vi "FPGA - Download (ECAT).vi"(8 "error in (no error)":errorcluster, 11 "Node Ptr":u64 format="%.0x") -> (0 "error out":errorcluster)   [LabVIEW 2016, in "Scan Engine Custom Device.lvlib"]
uses:
  Scan Engine Custom Device.lvlib
  Type Defs/FPGA Target.ctl
panel:
  in  "Tag":string
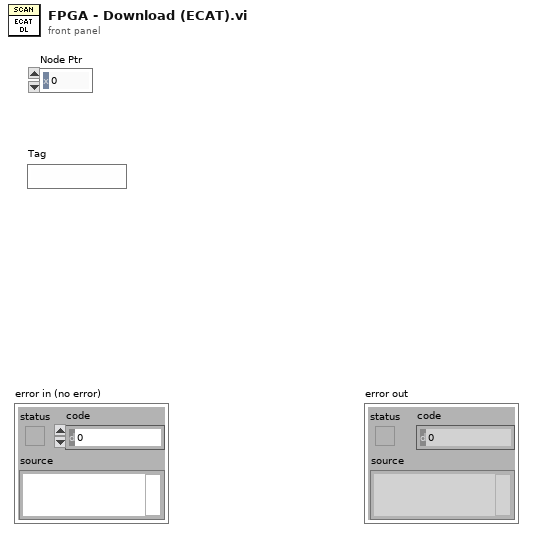
[diagram p1: front panel]
types:
  T1 = typedef "Scan Engine Custom Device.lvlib/FPGA Target.ctl" = enum16{"Local", "EtherCAT"}
  T2 = typedef "Custom Device API.lvlib/Custom Device Item Ref.ctl" = u64
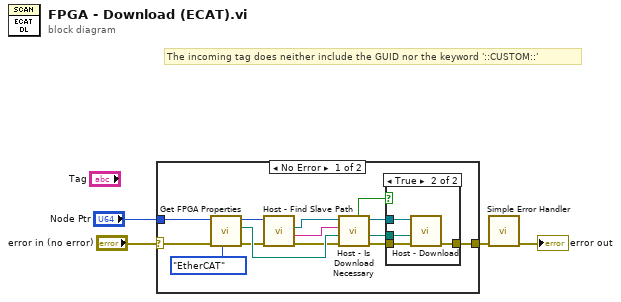
[diagram p0: block diagram]
diagram:
  # "The incoming tag does neither include the GUID nor the keyword '::CUSTOM::'"
  n1 = case shown="No Error" "error in (no error)" {
    selector: "error in (no error)" -> [w7 w24]
    tunnel: "Node Ptr" -> [w5 _]
    tunnel: [w6 w24] -> w2
    frame No Error {
      n2 = call "Get FPGA Properties.vi"("FPGA Target"=FPGA_Target."EtherCAT", "error in (no error)"=w7, "Item Ref in"=w5) -> ("error out"=w11:errorcluster, "Bitfile Path"=w13:path, "Item Ref out"=w12:T2)  [unwired: 5 in, 1 out]
      n3 = call "Host - Find Slave Path.vi"("error in (no error)"=w11, "Item Ref in"=w12) -> ("error out"=w9:errorcluster, "Target IP Address"=w10:string, "Slave Ref"=w8:refnum<k21>)  [unwired: 6 in, 1 out]
      n4 = call "Host - Is Download Necessary.vi"("Error In (no error)"=w9, "bitfile path in"=w13, "Target IP Address in"=w10, "Slave Ref in"=w8) -> ("error out"=w15:errorcluster, "bitfile path out"=w16:path, "Slave Ref out"=w17:refnum<k21>, "is download necessary?"=w14:bool)  [unwired: 3 in, 1 out]
      n5 = case shown="True" w14 {
        tunnel: w15 -> [w19 w23]
        tunnel: w16 -> [_ w22]
        tunnel: w17 -> [_ w21]
        tunnel: [w19 w20] -> w6
        frame False {
        }
        frame True {
          n6 = call "Host - Download.vi"("Error In (no error)"=w23, "bitfile path in"=w22, "Slave Ref in"=w21) -> ("error out"=w20:errorcluster)  [unwired: 6 in, 2 out]
        }
      }
    }
    frame Error {
    }
  }
  n7 = call <vilib>:"Simple Error Handler.vi"("error in (no error)"=w2) -> ("error out"=→"error out":errorcluster)  [unwired: 4 in, 4 out]
